vi "Anything to String Converter.vi"(1 "anything":variant) -> (0 "String":string)   [LabVIEW 2017, in "MU_3SL_interface.lvlib"]
doc: "Converts any data type into a string. If the data consists of \nmultiple values, they are separated with a comma.\nArrays are delimited by round brackets.\nCluster are delimited by square brackets."
uses:
  MU_3SL_interface.lvlib
  <vilib>/Utility/Data Type/NI_Data Type.lvlib
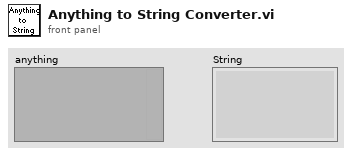
[diagram p1: front panel]
types:
  T1 = typedef "NI_Data Type.lvlib/Data Type.ctl" = enum8{"Invalid Type", "Void", "I8", "I16", "I32", "I64", "U8", "U16", "U32", "U64", "Single Float", "Double Float", "Extended Float", "Single Complex", "Double Complex", "Extended Complex", "Enum U8", "Enum U16", "Enum U32", "Enum U64", "Single Float With Unit", "Double Float With Unit", "Extended Float With Unit", "Single Complex with Unit", "Double Complex with Unit", "Extended Complex with Unit", "Boolean", "String", "Path", "Picture", "Tag", "Array", "Cluster", "Variant", "LV Variant", "Waveform", "Timestamp", "Digital Waveform", "Digital Data", "ExpressData", "Refnum", "External Data", "VI", "Poly VI", "LabVIEW Class Instance", "Fixed Point"}
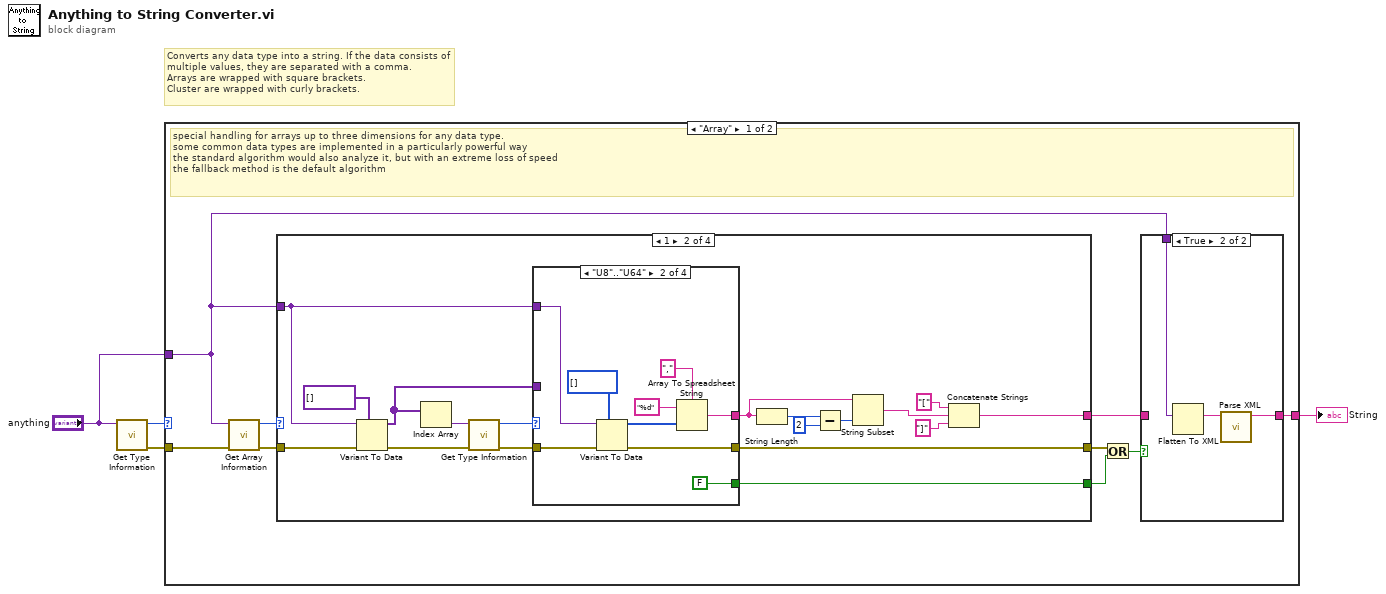
[diagram p0: block diagram]
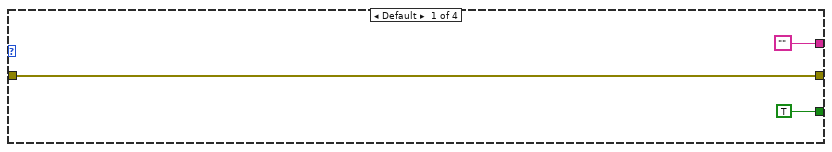
[diagram p2: hidden frame]
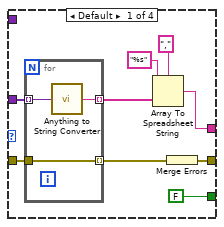
[diagram p3: hidden frame]
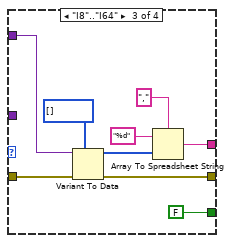
[diagram p4: hidden frame]
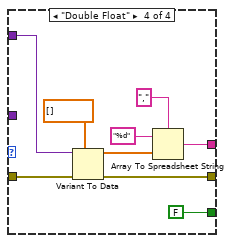
[diagram p5: hidden frame]
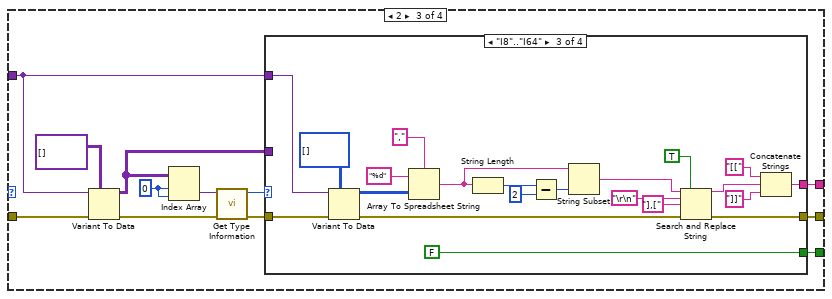
[diagram p6: hidden frame]
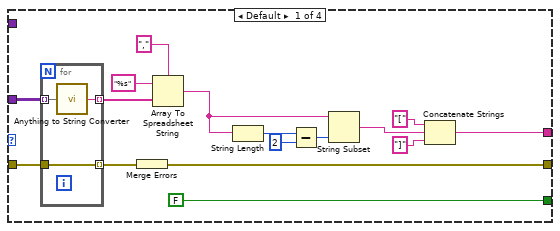
[diagram p7: hidden frame]
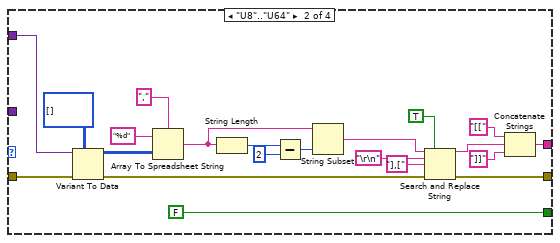
[diagram p8: hidden frame]
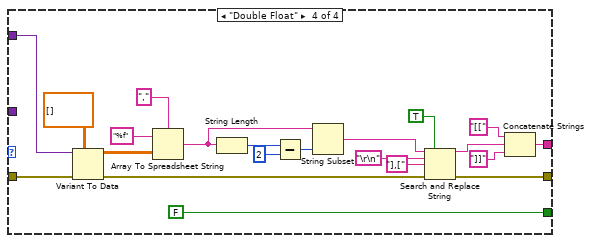
[diagram p9: hidden frame]
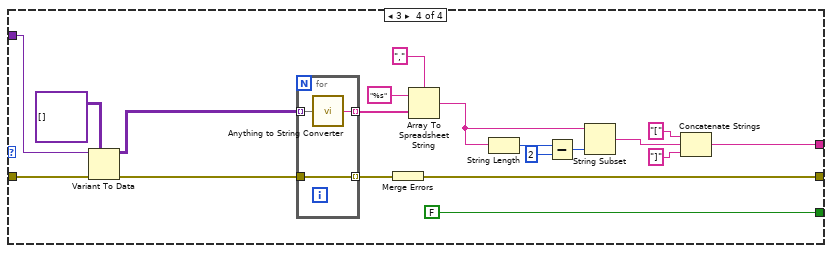
[diagram p10: hidden frame]
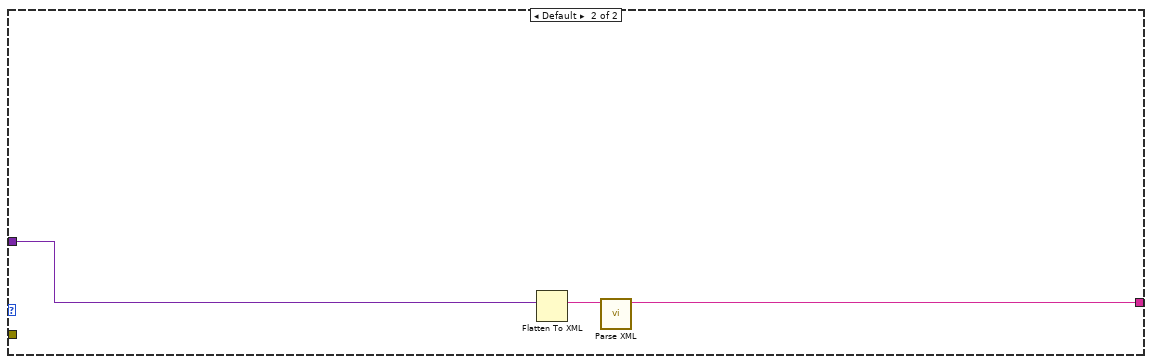
[diagram p12: hidden frame]
diagram:
  # "Converts any data type into a string. If the data consists of \nmultiple values, they are separated with a comma.\nArrays are wrapped with square brackets.\nCluster are wrapped with curly brackets."
  n1 = call <vilib>:"Get Type Information.vi"("Variant"="anything") -> ("error out"=w2:errorcluster, "Type"=w1:T1)  [unwired: 6 in, 3 out]
  n2 = case shown="\"Array\"" w1 {
    tunnel: [w13 w196] -> w4
    tunnel: w2 -> [w7 _]
    tunnel: "anything" -> [w10 w194]
    frame "Array" {
      # "special handling for arrays up to three dimensions for any data type.\nsome common data types are implemented in a particularly powerful way\nthe standard algorithm would also analyze it, but with an extreme loss of speed\nthe fallback method is the default algorithm"
      n3 = call <vilib>:"Get Array Information.vi"("error in (no error)"=w7, "Variant"=w10) -> ("error out"=w6:errorcluster, "Number of Dimensions"=w5:i32)  [unwired: 6 in, 2 out]
      n4 = case shown="1" w5 {
        tunnel: w10 -> [_ w29 w80 w185]
        tunnel: [w14 w28 w76 w181] -> w9
        tunnel: [TRUE w31 w79 FALSE] -> w8
        tunnel: ["" w25 w75 w180] -> w12
        tunnel: w6 -> [w14 w24 w78 w183]
        frame Default {
        }
        frame 1 {
          n5 = Variant To Data(error in=w24, type=variant[] [] ("anything"), Variant=w29) -> (data=w18:variant[], error out=w33:errorcluster)
          n6 = Index Array(array=w18) -> (element=w32:variant)  [unwired: 1 in]
          n7 = call <vilib>:"Get Type Information.vi"("error in (no error)"=w33, "Variant"=w32) -> ("error out"=w30:errorcluster, "Type"=w17:T1)  [unwired: 5 in, 3 out]
          n8 = case shown="\"U8\"..\"U64\"" w17 {
            tunnel: [FALSE FALSE FALSE FALSE] -> w31
            tunnel: w30 -> [w41 w54 w63 w72]
            tunnel: w29 -> [_ w53 w62 w71]
            tunnel: [w35 w48 w57 w66] -> w19
            tunnel: [w40 w47 w56 w65] -> w28
            tunnel: w18 -> [w39 _ _ _]
            frame Default {
              n9 = for {
                tunnel: [w46] -> w42 mode=indexing
                tunnel: w41 -> [w46]
                tunnel: w39 -> [w45] mode=indexing
                tunnel: [w44] -> w37 mode=indexing
                n10 = call "Anything to String Converter.vi"("anything"=w45) -> ("String"=w44:string)
              }
              n11 = Array To Spreadsheet String(delimiter (Tab)=",", array=w37, 3:"%s" ("format string")) -> (spreadsheet string=w35:string)
              n12 = Merge Errors(w42) -> (w40:errorcluster)
            }
            frame "U8".."U64" {
              n13 = Variant To Data(error in=w54, type=u64[] [], Variant=w53) -> (data=w51:u64[], error out=w47:errorcluster)
              n14 = Array To Spreadsheet String(delimiter (Tab)=",", array=w51, 3:"%d" ("format string")) -> (spreadsheet string=w48:string)
            }
            frame "I8".."I64" {
              n15 = Variant To Data(error in=w63, type=i64[] [], Variant=w62) -> (data=w60:i64[], error out=w56:errorcluster)
              n16 = Array To Spreadsheet String(delimiter (Tab)=",", array=w60, 3:"%d" ("format string")) -> (spreadsheet string=w57:string)
            }
            frame "Double Float" {
              n17 = Variant To Data(error in=w72, type=dbl[] [], Variant=w71) -> (data=w69:dbl[], error out=w65:errorcluster)
              n18 = Array To Spreadsheet String(delimiter (Tab)=",", array=w69, 3:"%d" ("format string")) -> (spreadsheet string=w66:string)
            }
          }
          n19 = String Length(string=w19) -> (length=w23:i32)
          n20 = Subtract(x=w23, y=2) -> (x-y=w22:i32)
          n21 = String Subset(string=w19, length (rest)=w22) -> (substring=w20:string)  [unwired: 1 in]
          n22 = Concatenate Strings("[" ("replace string (\"\")"), w20, "]" ("replace string (\"\")")) -> (w25:string)
        }
        frame 2 {
          w84 = 0 ("index (row)")
          n23 = Variant To Data(error in=w78, type=variant[][] [] ("anything"), Variant=w80) -> (data=w77:variant[][], error out=w82:errorcluster)
          n24 = Index Array(array=w77, index (row)=w84, index (col)=w84) -> (element=w81:variant)
          n25 = call <vilib>:"Get Type Information.vi"("error in (no error)"=w82, "Variant"=w81) -> ("error out"=w83:errorcluster, "Type"=w74:T1)  [unwired: 5 in, 3 out]
          n26 = case shown="\"I8\"..\"I64\"" w74 {
            tunnel: [FALSE FALSE FALSE FALSE] -> w79
            tunnel: w83 -> [w100 w124 w145 w166]
            tunnel: w80 -> [_ w123 w144 w165]
            tunnel: [w86 w108 w133 w150] -> w75
            tunnel: [w98 w105 w130 w151] -> w76
            tunnel: w77 -> [w97 _ _ _]
            frame Default {
              n27 = for {
                tunnel: w100 -> [w104]
                tunnel: [w104] -> w99 mode=indexing
                tunnel: w97 -> [w103] mode=indexing
                tunnel: [w102] -> w95 mode=indexing
                n28 = call "Anything to String Converter.vi"("anything"=w103) -> ("String"=w102:string)
              }
              n29 = Merge Errors(w99) -> (w98:errorcluster)
              n30 = Array To Spreadsheet String(delimiter (Tab)=",", array=w95, 3:"%s" ("format string")) -> (spreadsheet string=w87:string)
              n31 = String Length(string=w87) -> (length=w93:i32)
              n32 = Subtract(x=w93, y=2) -> (x-y=w92:i32)
              n33 = String Subset(string=w87, length (rest)=w92) -> (substring=w91:string)  [unwired: 1 in]
              n34 = Concatenate Strings("[" ("replace string (\"\")"), w91, "]" ("replace string (\"\")")) -> (w86:string)
            }
            frame "U8".."U64" {
              n35 = Variant To Data(error in=w124, type=u64[][] [], Variant=w123) -> (data=w121:u64[][], error out=w106:errorcluster)
              n36 = Array To Spreadsheet String(delimiter (Tab)=",", array=w121, 3:"%d" ("format string")) -> (spreadsheet string=w107:string)
              n37 = String Length(string=w107) -> (length=w118:i32)
              n38 = Subtract(x=w118, y=2) -> (x-y=w117:i32)
              n39 = String Subset(string=w107, length (rest)=w117) -> (substring=w116:string)  [unwired: 1 in]
              n40 = Search and Replace String(replace all?=TRUE ("replace all? (F)"), input string=w116, search string="\r\n", replace string="],[" ("replace string (\"\")"), error in=w106) -> (result string=w115:string, error out=w105:errorcluster)  [unwired: 3 in, 2 out]
              n41 = Concatenate Strings("[[" ("replace string (\"\")"), w115, "]]" ("replace string (\"\")")) -> (w108:string)
            }
            frame "I8".."I64" {
              n42 = Variant To Data(error in=w145, type=i64[][] [], Variant=w144) -> (data=w142:i64[][], error out=w131:errorcluster)
              n43 = Array To Spreadsheet String(delimiter (Tab)=",", array=w142, 3:"%d" ("format string")) -> (spreadsheet string=w132:string)
              n44 = String Length(string=w132) -> (length=w139:i32)
              n45 = Subtract(x=w139, y=2) -> (x-y=w138:i32)
              n46 = String Subset(string=w132, length (rest)=w138) -> (substring=w137:string)  [unwired: 1 in]
              n47 = Search and Replace String(replace all?=TRUE ("replace all? (F)"), input string=w137, search string="\r\n", replace string="],[" ("replace string (\"\")"), error in=w131) -> (result string=w136:string, error out=w130:errorcluster)  [unwired: 3 in, 2 out]
              n48 = Concatenate Strings("[[" ("replace string (\"\")"), w136, "]]" ("replace string (\"\")")) -> (w133:string)
            }
            frame "Double Float" {
              n49 = Variant To Data(error in=w166, type=dbl[][] [], Variant=w165) -> (data=w163:dbl[][], error out=w154:errorcluster)
              n50 = Array To Spreadsheet String(delimiter (Tab)=",", array=w163, 3:"%f" ("format string")) -> (spreadsheet string=w149:string)
              n51 = String Length(string=w149) -> (length=w158:i32)
              n52 = Subtract(x=w158, y=2) -> (x-y=w157:i32)
              n53 = String Subset(string=w149, length (rest)=w157) -> (substring=w156:string)  [unwired: 1 in]
              n54 = Search and Replace String(replace all?=TRUE ("replace all? (F)"), input string=w156, search string="\r\n", replace string="],[" ("replace string (\"\")"), error in=w154) -> (result string=w155:string, error out=w151:errorcluster)  [unwired: 3 in, 2 out]
              n55 = Concatenate Strings("[[" ("replace string (\"\")"), w155, "]]" ("replace string (\"\")")) -> (w150:string)
            }
          }
        }
        frame 3 {
          n56 = Variant To Data(error in=w183, type=variant[][][] [] ("anything"), Variant=w185) -> (data=w182:variant[][][], error out=w168:errorcluster)
          n57 = for {
            tunnel: w168 -> [w189]
            tunnel: [w189] -> w179 mode=indexing
            tunnel: w182 -> [w188] mode=indexing
            tunnel: [w187] -> w177 mode=indexing
            n58 = call "Anything to String Converter.vi"("anything"=w188) -> ("String"=w187:string)
          }
          n59 = Merge Errors(w179) -> (w181:errorcluster)
          n60 = Array To Spreadsheet String(delimiter (Tab)=",", array=w177, 3:"%s" ("format string")) -> (spreadsheet string=w169:string)
          n61 = String Length(string=w169) -> (length=w175:i32)
          n62 = Subtract(x=w175, y=2) -> (x-y=w174:i32)
          n63 = String Subset(string=w169, length (rest)=w174) -> (substring=w173:string)  [unwired: 1 in]
          n64 = Concatenate Strings("[" ("replace string (\"\")"), w173, "]" ("replace string (\"\")")) -> (w180:string)
        }
      }
      n65 = Or(x=w9, y=w8) -> (x .or. y?=w11:bool)
      n66 = case shown="True" w11 {
        tunnel: [w190 w193] -> w13
        tunnel: w12 -> [w190 _]
        tunnel: w10 -> [_ w191]
        frame False {
        }
        frame True {
          n67 = Flatten To XML(anything=w191) -> (xml string=w192:string)
          n68 = call "Parse XML.vi"("XML String Input"=w192) -> ("Parsed Value"=w193:string)  [unwired: 9 in, 1 out]
        }
      }
    }
    frame Default {
      n69 = Flatten To XML(anything=w194) -> (xml string=w195:string)
      n70 = call "Parse XML.vi"("XML String Input"=w195) -> ("Parsed Value"=w196:string)  [unwired: 9 in, 1 out]
    }
  }
  "String" <- w4
